vi "Create Value.vi"(8 "error in (no error)":errorcluster, 11 "NT Scalar in":refnum<class "NT Scalar.lvclass">) -> (0 "error out":errorcluster, 2 "PV Data out":refnum<class "PV Data.lvclass">, 3 "NT Scalar out":refnum<class "NT Scalar.lvclass">)   [LabVIEW 2020, in "PV Access.lvlib" / "PV Data.lvlib" / "NT Scalar.lvclass"]
uses:
  NT Scalar.lvclass
  C:/Users/eyw68381/source/repos/pvaccess-labview/labview/source/PV Data/NT Base/NT Base.lvclass
  PV Data/PV Data.lvclass
  cd2aede2-f021-44bb-be08-44984694ca73.vi
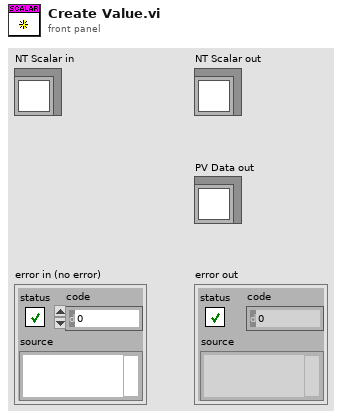
[diagram p1: front panel]
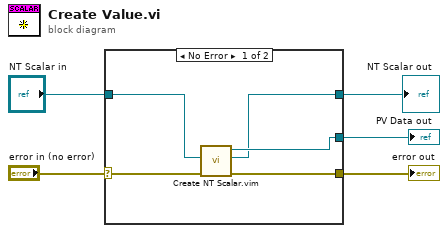
[diagram p0: block diagram]
diagram:
  n1 = case shown="No Error" "error in (no error)" {
    selector: "error in (no error)" -> [w6 w12]
    tunnel: [w10 w12] -> w3
    tunnel: [w7 w11] -> w2
    tunnel: "NT Scalar in" -> [w8 w11]
    tunnel: [w9 _] -> w1
    frame No Error {
      n2 = call "Create NT Scalar.vim"("error in (no error)"=w6, "initial value"=w8) -> ("error out"=w10:errorcluster, "value out"=w7:refnum<class "NT Scalar.lvclass">, "PV Data out"=w9:refnum<class "PV Data.lvclass">)  [unwired: 6 in, 1 out]
    }
    frame Error {
    }
  }
  "error out" <- w3
  "NT Scalar out" <- w2
  "PV Data out" <- w1
